vi "Main.vi"(8 "error in":errorcluster, 11 "BEEP in":refnum<class "BEEP.lvclass">) -> (0 "error out":errorcluster, 3 "BEEP out":refnum<class "BEEP.lvclass">)   [LabVIEW 2024, in "BEEP.lvclass"]
doc: "The <b>Queued Message Handler</b> of the Worker that owns this VI."
uses:
  BEEP.lvclass
  rqp_Beep.ctl
  BEEP.lvclass/BEEP.ctl
  <vilib>/Python/Open Venv Python Session.vi
  <vilib>/addons/_Workers/Library/Classes/Message Queue/Message Queue.lvclass
panel:
  in  "bBeep":bool
  in  "Duration [ms]":dbl
  in  "Frecency [Hz]":dbl
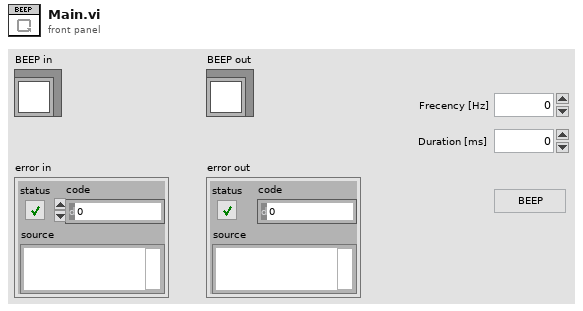
[diagram p1: front panel]
types:
  T1 = typedef "BEEP.lvclass/rqp_Beep.ctl" = cluster{"Frecency [Hz]":u32, "Duration [ms]":u32}
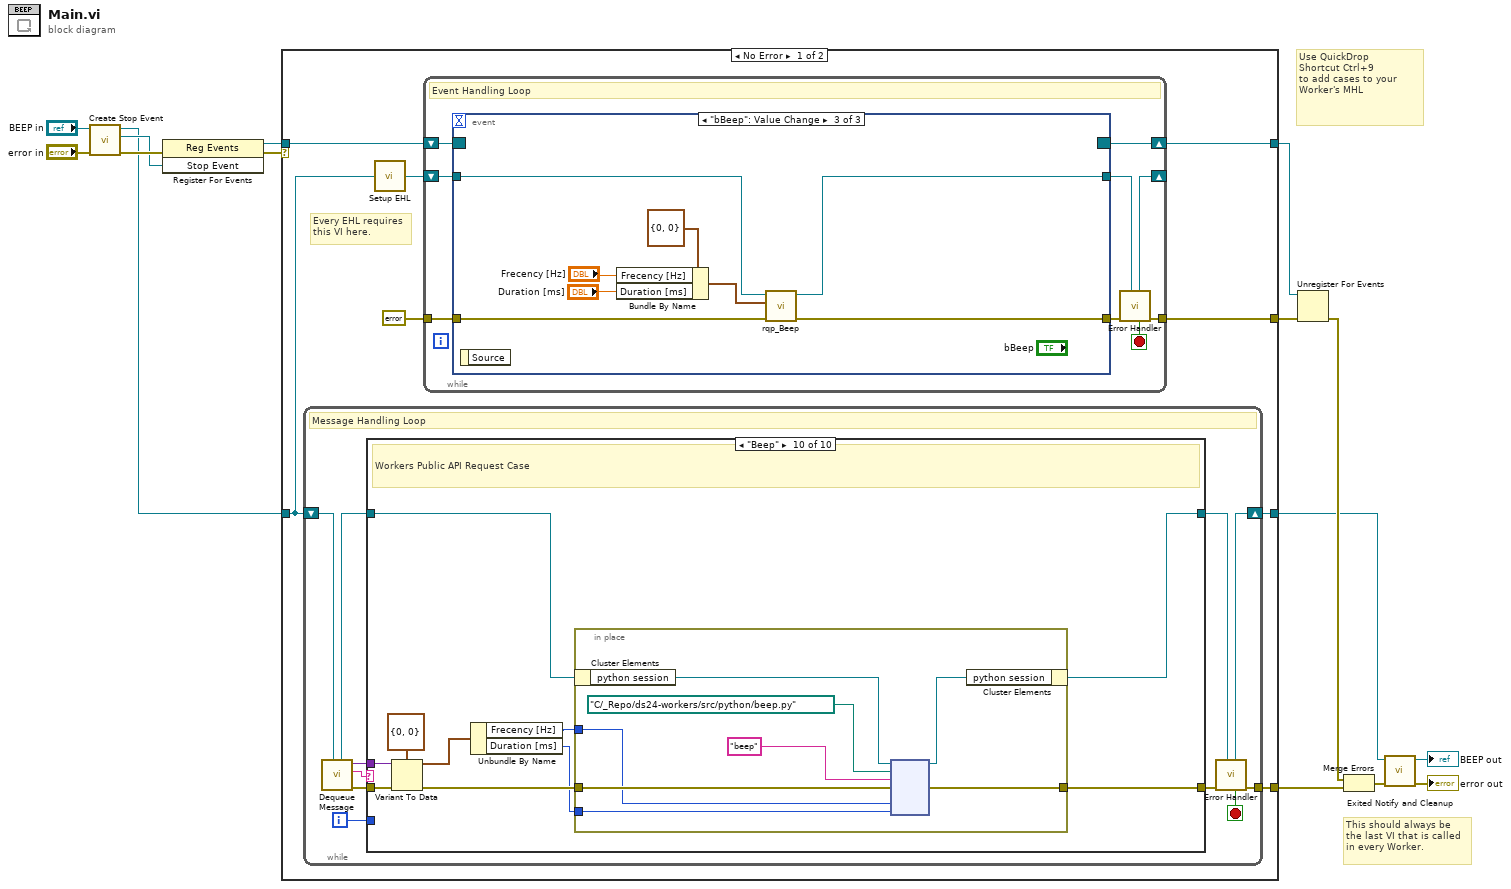
[diagram p0: block diagram]
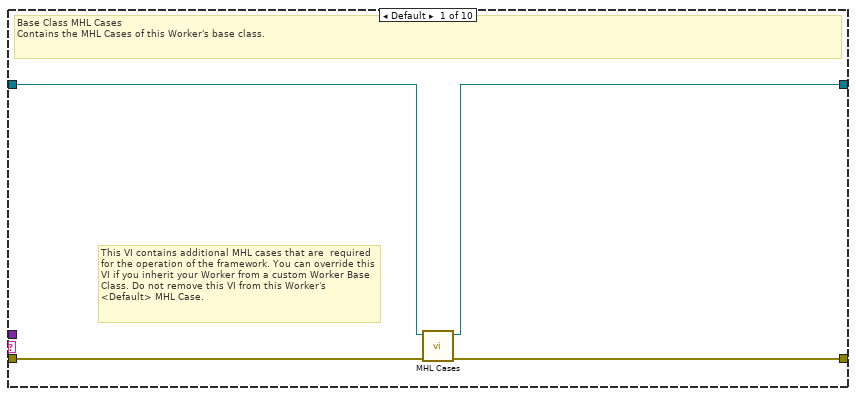
[diagram p2: hidden frame]
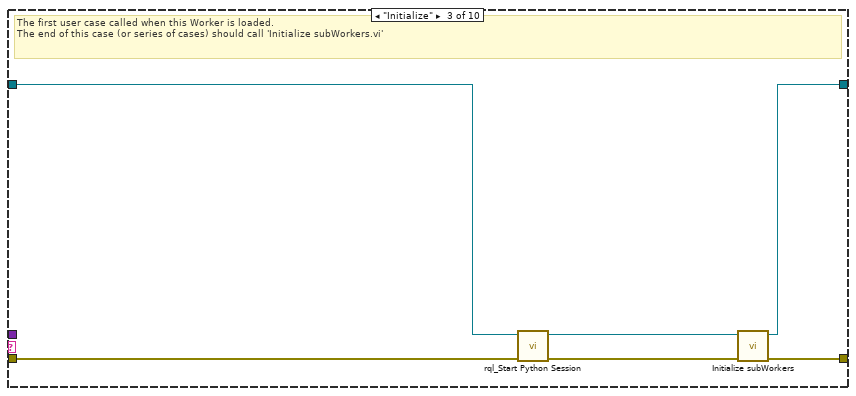
[diagram p4: hidden frame]
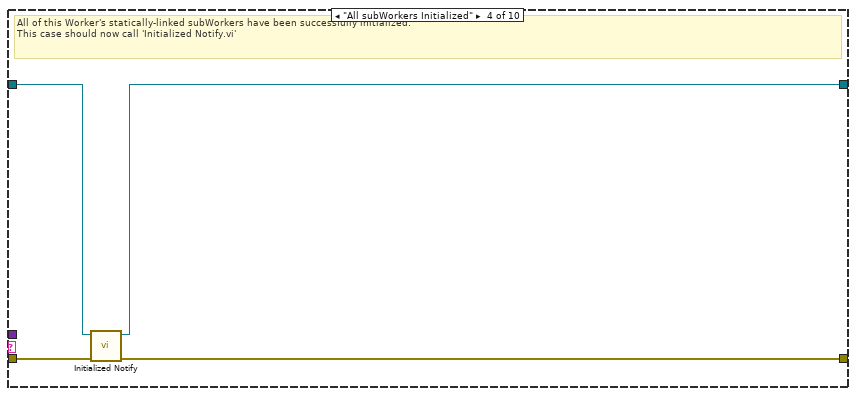
[diagram p5: hidden frame]
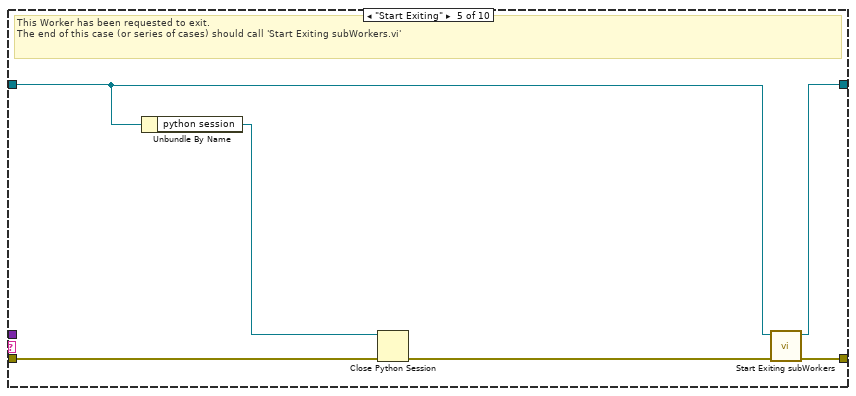
[diagram p6: hidden frame]
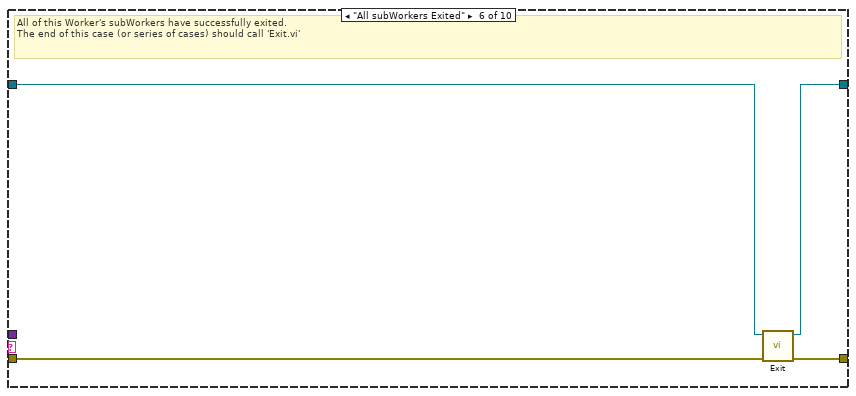
[diagram p7: hidden frame]
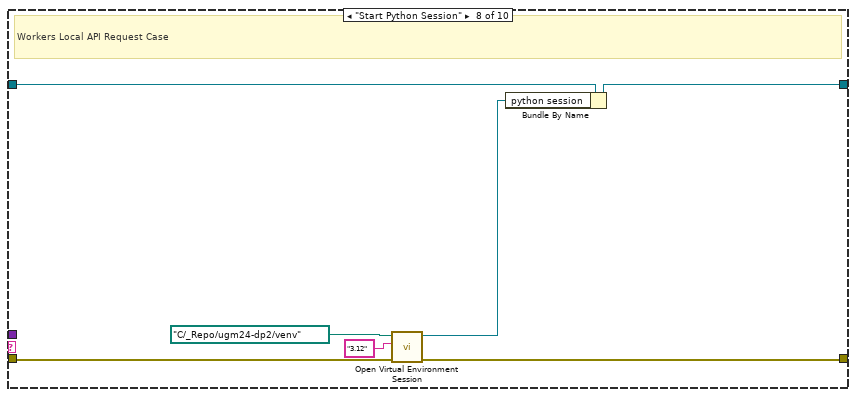
[diagram p9: hidden frame]
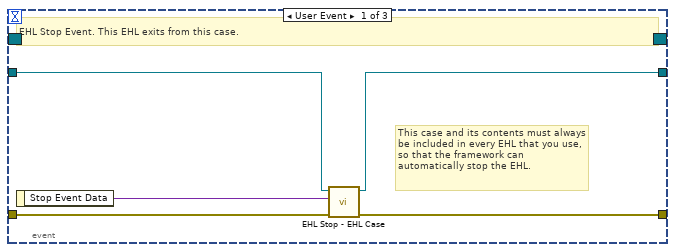
[diagram p11: hidden frame]
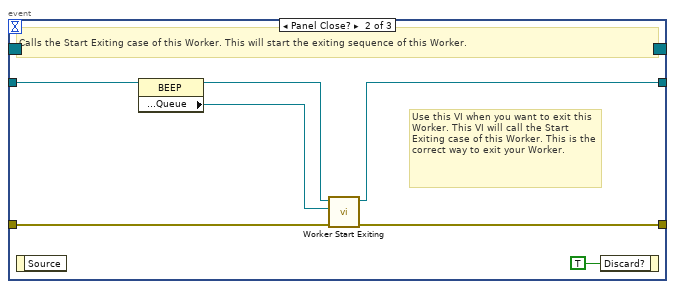
[diagram p12: hidden frame]
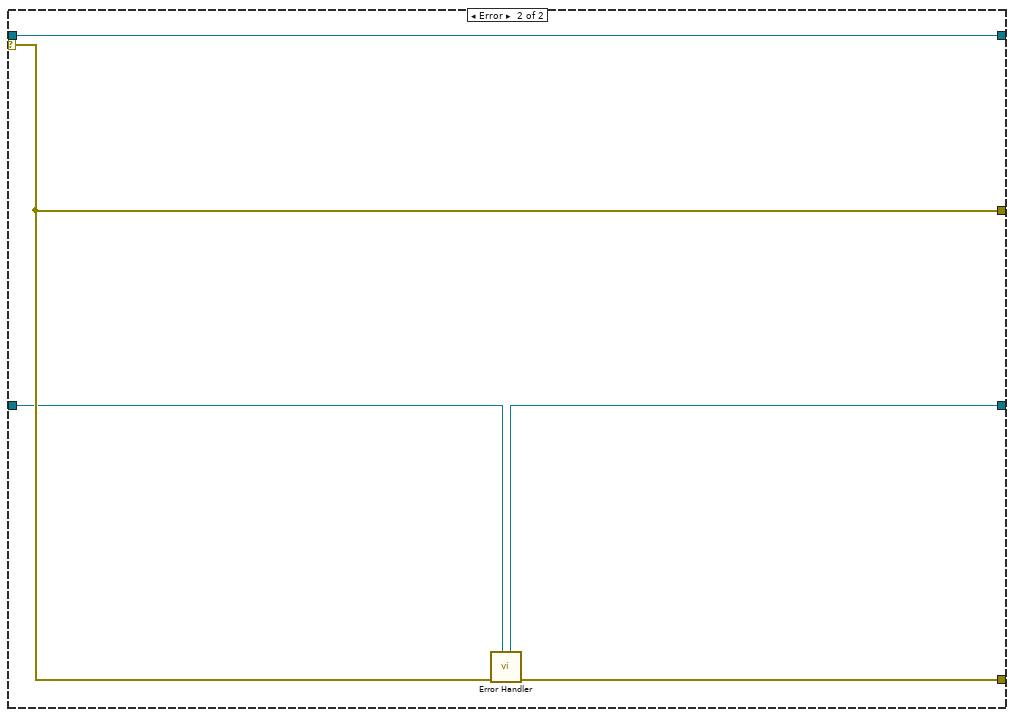
[diagram p13: hidden frame]
diagram:
  # "Use QuickDrop\nShortcut Ctrl+9\nto add cases to your\nWorker's MHL"
  # "This should always be the last VI that is called in every Worker."
  n1 = call-dynamic "Create Stop Event.vi"("error in"="error in", "Worker"="BEEP in") -> ("error out"=w10:errorcluster, "Stop Event"=w7:refnum<user-event>, "Worker out"=w4:refnum<class "BEEP.lvclass">)  [unwired: 7 in]
  n2 = register-events(error in=w10, w7) -> (reference out=w9:refnum<event-registration>, error out=w1:errorcluster)  [unwired: 1 in]
  n3 = case shown="No Error" w1 {
    tunnel: w4 -> [w18 w120]
    tunnel: [w16 w121] -> w8
    tunnel: w9 -> [w23 w122]
    tunnel: [w20 w123] -> w14
    tunnel: [w22 w122] -> w13
    tunnel: [w17 w119] -> w11
    selector: w1 -> [_ w123]
    frame No Error {
      # "Every EHL requires\nthis VI here."
      n4 = while {
        shift-right: [w32] -> w17
        shift-left: w18 -> [w34]
        tunnel: [w33] -> w16
        i -> [w25]
        stop <- w26 stop-if-true
        # "Message Handling Loop"
        n5 = call-dynamic "Dequeue Message.vi"("Worker"=w34) -> ("error out"=w31:errorcluster, "Case out"=w27:string, "Data out"=w24:variant, "Worker out"=w29:refnum<class "BEEP.lvclass">)  [unwired: 6 in, 1 out]
        n6 = case "Worker MHL Case Structure (DO NOT CHANGE LABEL NAME)" shown="\"Beep\"" w27 {
          tunnel: w31 -> [w38 w39 w41 w48 w54 w60 w62 w66 w71 w81]
          tunnel: [w37 w39 w46 w47 w56 w59 w62 w65 w71 w76] -> w30
          tunnel: w29 -> [w36 w40 w42 w50 w53 w58 w61 w69 w70 w72]
          tunnel: [w35 w40 w45 w49 w55 w57 w61 w64 w70 w73] -> w28
          tunnel: w25 -> [_ _ _ _ _ _ _ _ _ _]
          tunnel: w24 -> [_ _ _ _ _ _ _ _ _ w78]
          frame Default {
            # "This VI contains additional MHL cases that are  required for the operation of the framework. You can override this VI if you inherit your Worker from a custom Worker Base Class. Do not remove this VI from this Worker's <Default> MHL Case."
            # "Base Class MHL Cases\nContains the MHL Cases of this Worker's base class."
            n7 = call-dynamic "MHL Cases.vi"("error in"=w38, "Worker in"=w36) -> ("error out"=w37:errorcluster, "Worker out"=w35:refnum<class "BEEP.lvclass">)  [unwired: 8 in]
          }
          frame "------------ FRAMEWORK CASES -----------" {
            # "Start of Workers Framework Cases"
          }
          frame "Initialize" {
            # "The first user case called when this Worker is loaded.\nThe end of this case (or series of cases) should call 'Initialize subWorkers.vi'"
            n8 = call "rql_Start Python Session.vi"("error in"=w41, "CPU Percent in"=w42) -> ("error out"=w44:errorcluster, "dup CPU Percent out"=w43:refnum<class "BEEP.lvclass">)  [unwired: 8 in]
            n9 = call-dynamic "Initialize subWorkers.vi"("error in"=w44, "Worker"=w43) -> ("error out"=w46:errorcluster, "dup Worker out"=w45:refnum<class "BEEP.lvclass">)  [unwired: 8 in]
          }
          frame "All subWorkers Initialized" {
            # "All of this Worker's statically-linked subWorkers have been successfully initialized.\nThis case should now call 'Initialized Notify.vi'"
            n10 = call-dynamic "Initialized Notify.vi"("error in"=w48, "Worker"=w50) -> ("error out"=w47:errorcluster, "dup Worker out"=w49:refnum<class "BEEP.lvclass">)  [unwired: 8 in]
          }
          frame "Start Exiting" {
            # "This Worker has been requested to exit. \nThe end of this case (or series of cases) should call 'Start Exiting subWorkers.vi'"
            n11 = Unbundle By Name(w53) -> ("python session"=w51:refnum<k35>)
            n12 = Close Python Session(session in=w51, error in=w54) -> (11:w52:errorcluster)
            n13 = call-dynamic "Start Exiting subWorkers.vi"("error_in"=w52, "Worker"=w53) -> ("error out"=w56:errorcluster, "dup Worker out"=w55:refnum<class "BEEP.lvclass">)  [unwired: 8 in]
          }
          frame "All subWorkers Exited" {
            # "All of this Worker's subWorkers have successfully exited. \nThe end of this case (or series of cases) should call 'Exit.vi'"
            n14 = call-dynamic "Exit.vi"("error_in"=w60, "Worker"=w58) -> ("error out"=w59:errorcluster, "dup Worker out"=w57:refnum<class "BEEP.lvclass">)  [unwired: 8 in]
          }
          frame "------------- LOCAL API CASES -------------" {
            # "Start of Workers Local API Cases"
          }
          frame "Start Python Session" {
            # "Workers Local API Request Case"
            n15 = call-poly <vilib>:"Open Virtual Environment Session.vi"("error in (no error)"=w66, "Python version"="3.12", "Env path"=path "C:/_Repo/ugm24-dp2/venv") -> ("error out"=w65:errorcluster, "session out"=w63:refnum<k35>)  [unwired: 7 in]
            n16 = Bundle By Name(cluster=w69, "python session"=w63) -> (w64:refnum<class "BEEP.lvclass">)
          }
          frame "------------- PUBLIC API CASES -------------" {
            # "Start of Workers Public API Cases"
          }
          frame "Beep" {
            # "Workers Public API Request Case"
            n17 = Variant To Data(error in=w81, type=T1 {"Frecency [Hz]"=0, "Duration [ms]"=0} ("Data"), Variant=w78) -> (data=w77:T1, error out=w80:errorcluster)
            n18 = Unbundle By Name(w77) -> ("Frecency [Hz]"=w75:u32, "Duration [ms]"=w74:u32)
            n19 = in-place {
              in-place-border: w80 -> [w89]
              in-place-border: [w88] -> w76
              in-place-border: w75 -> [w87]
              in-place-border: w74 -> [w86]
              n20 = in-place-cluster #1(w72) -> ("python session"=w85:refnum<k35>)
              n21 = node(w85, path "C:/_Repo/ds24-workers/src/python/beep.py" ("module path"), "beep" ("function name"), w89, w87, w86) -> (w84:refnum<k35>, w88:errorcluster)  [unwired: 4 in, 2 out]
              n22 = in-place-cluster #1("python session"=w84) -> (w73:refnum<class "BEEP.lvclass">)
            }
          }
        }
        n23 = call-dynamic "Error Handler.vi"("Worker"=w28, "error_in"=w30) -> ("error out"=w33:errorcluster, "Stop Loop"=w26:bool, "Worker out"=w32:refnum<class "BEEP.lvclass">)  [unwired: 7 in]
      }
      n24 = call-dynamic "Setup EHL.vi"("Worker"=w18) -> ("Worker out"=w19:refnum<class "BEEP.lvclass">)  [unwired: 14 in]
      n25 = while "Event Handling Loop" {
        shift-right: [w98] -> w22
        shift-left: w23 -> [w97]
        tunnel: [w93] -> w20
        tunnel: errorcluster {"status"=FALSE, "code"=0, "source"=""} ("error constant") -> [w95]
        shift-right: [w91] -> _
        shift-left: w19 -> [w96]
        stop <- w90 stop-if-true
        # "Event Handling Loop"
        n26 = event shown="[2] \"bBeep\": Value Change" {
          selector: w97 -> [_ _ _]
          dyn-events: [_ _ _] -> w98
          timeout: _ -> [_ _ _]
          tunnel: [w102 w109 w117] -> w94
          tunnel: w95 -> [w103 w108 w118]
          tunnel: w96 -> [w101 w107 w116]
          tunnel: [w100 w106 w115] -> w92
          event User Event {
            # "This case and its contents must always be included in every EHL that you use, so that the framework can automatically stop the EHL."
            # "EHL Stop Event. This EHL exits from this case."
            n27 = event-data() -> ("Stop Event Data"=w99:variant)  [unwired: 1 in]
            n28 = call-dynamic "EHL Stop - EHL Case.vi"("error in"=w103, "Stop Event Data"=w99, "Worker"=w101) -> ("error out"=w102:errorcluster, "Worker out"=w100:refnum<class "BEEP.lvclass">)  [unwired: 7 in]
          }
          event Panel Close? {
            # "Use this VI when you want to exit this Worker. This VI will call the Start Exiting case of this Worker. This is the correct way to exit your Worker."
            # "Calls the Start Exiting case of this Worker. This will start the exiting sequence of this Worker."
            n29 = event-data() -> ()  [unwired: 1 in, 1 out]
            n30 = property class="BEEP"(reference=w107) -> (reference out=w105:refnum<class "BEEP.lvclass">, "Accessors:Read:Public API:Queue"=w104:refnum<class "Message Queue.lvclass">)  [unwired: 1 in, 1 out]
            n31 = call-dynamic "Worker Start Exiting.vi"("error_in"=w108, "Message Queue"=w104, "Worker"=w105) -> ("error out"=w109:errorcluster, "dup Worker out"=w106:refnum<class "BEEP.lvclass">)  [unwired: 7 in]
            n32 = event-data("Discard?"=TRUE) -> ()  [unwired: 1 in, 1 out]
          }
          event "bBeep": Value Change {
            n33 = event-data() -> ()  [unwired: 1 in, 1 out]
            n34 = Bundle By Name(cluster=T1 {"Frecency [Hz]"=0, "Duration [ms]"=0} ("Data in"), "Frecency [Hz]"="Frecency [Hz]", "Duration [ms]"="Duration [ms]") -> (w113:T1)
            n35 = call "rqp_Beep.vi"("error in"=w118, "Data in"=w113, "BEEP in"=w116) -> ("error out"=w117:errorcluster, "dup BEEP out"=w115:refnum<class "BEEP.lvclass">)  [unwired: 6 in, 1 out]
          }
        }
        n36 = call-dynamic "Error Handler.vi"("Worker"=w92, "error_in"=w94) -> ("error out"=w93:errorcluster, "Stop Loop"=w90:bool, "Worker out"=w91:refnum<class "BEEP.lvclass">)  [unwired: 7 in]
      }
    }
    frame Error {
      n37 = call-dynamic "Error Handler.vi"("Worker"=w120, "error_in"=w123) -> ("error out"=w121:errorcluster, "Worker out"=w119:refnum<class "BEEP.lvclass">)  [unwired: 7 in, 1 out]
    }
  }
  n38 = Unregister For Events(event registration refnum=w13, error in=w14) -> (error out=w15:errorcluster)
  n39 = Merge Errors(w15, w8) -> (w12:errorcluster)
  n40 = call-dynamic "Exited Notify and Cleanup.vi"("error_in"=w12, "Worker"=w11) -> ("error out"=→"error out":errorcluster, "dup Worker out"=→"BEEP out":refnum<class "BEEP.lvclass">)  [unwired: 8 in]
